vi "AB_User_Log_Source_Item.vi"(8 "error in (no error)":errorcluster, 9 "Version":string, 11 "sourcePath":path) -> (0 "error out":errorcluster)   [LabVIEW 2020]
uses:
  <vilib>/Utility/error.llb/whitespace.ctl
  <vilib>/AppBuilder/logging/AB_Log_File_Action.ctl
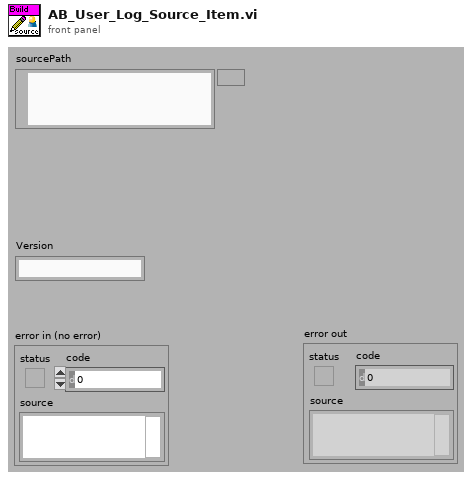
[diagram p1: front panel]
types:
  T1 = typedef "whitespace.ctl" = u16
  T2 = typedef "AB_Log_File_Action.ctl" = enum16{"write", "open", "close"}
  T3 = typedef "Librarian File Info Out.ctl" = cluster{"creation date":u32, "last mod date":u32, "type":string, "creator":string, "LV version":i32, "size":i32, "top level":bool}
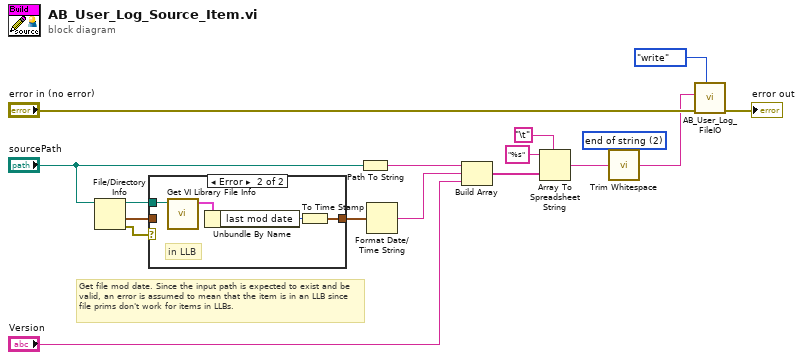
[diagram p0: block diagram]
diagram:
  w2 = T1 2 items=["both", "start of string", "end of string"] ("location (both)")
  # "Get file mod date. Since the input path is expected to exist and be valid, an error is assumed to mean that the item is in an LLB since file prims don't work for items in LLBs."
  n1 = File/Directory Info(path="sourcePath") -> (path out=w6:path, last mod=w4:timestamp, error out=w5:errorcluster)  [unwired: 1 in, 4 out]
  n2 = case shown="Error" w5 {
    tunnel: w6 -> [_ w22]
    tunnel: [w18 w19] -> w8
    tunnel: w4 -> [w18 _]
    frame No Error {
    }
    frame Error {
      # "in LLB"
      n3 = call <vilib>:"Get VI Library File Info.vi"("path"=w22) -> ("file information"=w21:T3)  [unwired: 1 in, 9 out]
      n4 = Unbundle By Name(w21) -> ("last mod date"=w20:u32)
      n5 = To Time Stamp(1:w20) -> (0:w19:timestamp)
    }
  }
  n6 = Path To String(path="sourcePath") -> (string=w15:string)
  n7 = Format Date/Time String(seconds (now)=w8) -> (date/time string=w14:string)  [unwired: 2 out]
  n8 = Build Array(w15, w14, "Version") -> (w12:string[])
  n9 = Array To Spreadsheet String(delimiter (Tab)="\t", array=w12, 3:"%s" ("format string")) -> (spreadsheet string=w10:string)
  n10 = call <vilib>:"Trim Whitespace.vi"("string"=w10, "location (both)"=w2) -> ("trimmed string"=w3:string)
  n11 = call <vilib>:"AB_User_Log_FileIO.vi"("fileAction"=AB_Log_File_Action."write", "error in (no error)"="error in (no error)", "data"=w3) -> ("error out"=→"error out":errorcluster)  [unwired: 2 in, 6 out]
